vi "UI Event-Settings-Value Change.vi"(8 "Error In":errorcluster, 11 "Root Panel Actor in":refnum<class "Root Panel Actor.lvclass">) -> (0 "Error Out":errorcluster, 3 "Root Panel Actor out":refnum<class "Root Panel Actor.lvclass">)   [LabVIEW 2021, in "Root Panel.lvlib" / "Root Panel Actor.lvclass"]
uses:
  Root Panel Actor.lvclass
  C:/Program Files (x86)/National Instruments/LabVIEW 2021/vi.lib/MGI/Panel Manager/Panel Actor/Panel Actor/Panel Actor.lvclass
  Modules/Settings Module/Settings Actor/Settings Actor.lvclass
  Root Panel Actor.lvclass/Root Panel Actor.ctl
  <vilib>/MGI/Panel Manager/Panel/Panel/Subpanel/Subpanel.lvclass
  C:/Program Files (x86)/National Instruments/LabVIEW 2021/vi.lib/MGI/Panel Manager/Panel/Panel/Panel.lvclass
  <vilib>/MGI/Panel Manager/Panel/Panel/Subpanel/Subpanel.vi
  <vilib>/MGI/Panel Manager/Panel Actor/Panel Actor/Panel Actor.lvclass
  <vilib>/MGI/Panel Manager/Panel/Panel.lvlib
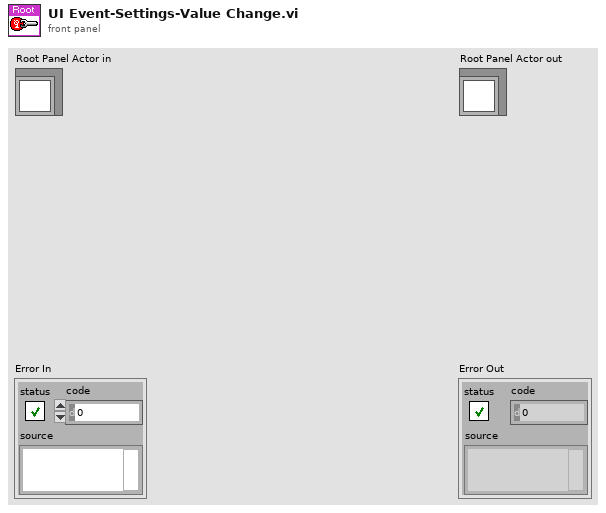
[diagram p1: front panel]
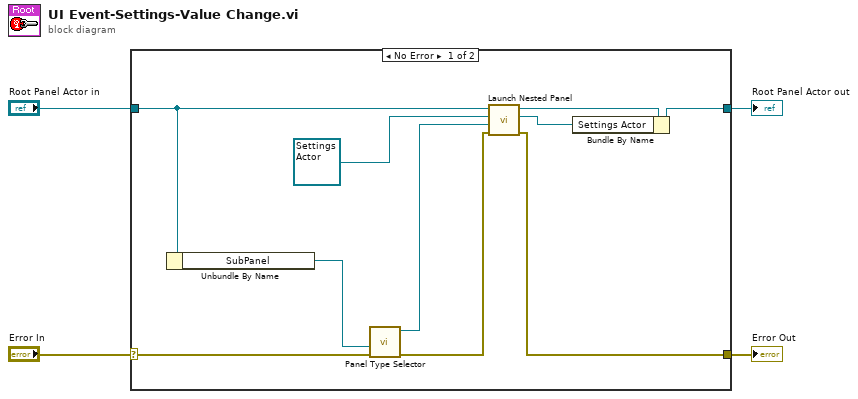
[diagram p0: block diagram]
diagram:
  n1 = case shown="No Error" "Error In" {
    selector: "Error In" -> [w10 w16]
    tunnel: [w11 w16] -> w3
    tunnel: [w13 w15] -> w1
    tunnel: "Root Panel Actor in" -> [w6 w15]
    frame No Error {
      n2 = Unbundle By Name(w6) -> ("SubPanel"=w5:refnum<vi>)
      n3 = call-poly <vilib>:"Panel Type Selector.vi"("Error In"=w10, "Sub Panel"=w5) -> ("Error Out"=w9:errorcluster, "Subpanel Out"=w8:refnum<class "Subpanel.lvclass">)  [unwired: 8 in]
      n4 = call <vilib>:"Launch Nested Panel.vi"("error in (no error)"=w9, "Panel"=w8, "Nested Panel Actor"=refnum<class "Settings Actor.lvclass"> refnum ("Settings Module.lvlib:Settings Actor.lvclass"), "Panel Actor in"=w6) -> ("error out"=w11:errorcluster, "Nested Actor's Enqueuer"=w12:refnum<class "Message Enqueuer.lvclass">, "Panel Actor out"=w14:refnum<class "Root Panel Actor.lvclass">)  [unwired: 4 in, 1 out]
      n5 = Bundle By Name(cluster=w14, "Settings Actor"=w12) -> (w13:refnum<class "Root Panel Actor.lvclass">)
    }
    frame Error {
    }
  }
  "Error Out" <- w3
  "Root Panel Actor out" <- w1
